vi "Read Power FIFO Direct Dispatch.vi"(7 "Release Lock":bool=TRUE, 8 "error in (no error)":errorcluster, 9 "Timeout (ms)":i32=100, 10 "Power Waveform In":T1, 11 "CIFTag in":refnum<class "CIFChannels.lvclass">) -> (0 "error out":errorcluster, 1 "timed out?":bool, 2 "Power Waveform Out":T1, 3 "CIFTag out":refnum<class "CIF_NIChn_Fifo_Power_DVR.lvclass">, 4 "Header":T2)   [LabVIEW 2021, in "CIF_NIChn_Fifo_Power_DVR.lvclass"]
uses:
  CIF_NIChn_Fifo_Power_DVR.lvclass
  D:/dev/CIF-LVCore/src/Channels/CIFChannels/CIFChannels.lvclass
  D:/dev/CIF-LVCore/src/Channels/CIF_NIChn/NIChn/CIF_NIChn.lvclass
  ChannelCommon/typedef/FIFO Header.ctl
  CIFChannels/CIFChannels.lvclass
  ChannelCommon/typedef/Datatype Power Waveform.ctl
  CIFChannels/CIFChannels.lvclass/CIFChannels.ctl
  NIChn/CIF_NIChn.lvclass/CIF_NIChn.ctl
  CIF_NIChn_Fifo_Power_DVR.lvclass/CIF_NIChn_Fifo_Power_DVR.ctl
  ChannelCommon/CIFFIFO/CIFfifo.lvclass/CIFfifo.ctl
  NIChn/Accessors/Read CIF Channel.vi
  NIChn/SubVIs/Check Disconnect.vi
  <vilib>/CIFChannels/Top Level/Read Variable Length U8 Array.vi
  NIChn/Accessors/Write CIF Channel.vi
  SubVIs/Unflatten.vi
  CIFChannels/Accessors/Read Channel State.vi
  CIFChannels/Accessors/Read Direction.vi
  CIFChannels/Accessors/Write Channel State.vi
  CIFChannels/Accessors/Read Disconnect Behavior.vi
  <vilib>/CIFChannels/Top Level/Read Variable Length U8 Array.vi/81056090-23cf-424a-a716-29db01c8ef1b.vi
  <vilib>/CIFChannels/Top Level/Read Variable Length U8 Array.vi/6610cd62-0a6d-4591-8fd4-6453482a4bc1.vi
  <vilib>/CIFChannels/Top Level/Read Variable Length U8 Array.vi/93d598b0-524b-4f76-9570-a74a86ef2c6f.vi
  ChannelCommon/CIFFIFO/Accessors/Write Timeout.vi
  ChannelCommon/CIFFIFO/Flatten/DVR Unflatten.vi
  ChannelCommon/CIFFIFO/Accessors/Read Header.vi
  ChannelCommon/CIFFIFO/Accessors/Write Header.vi
  <vilib>/CIFChannels/Top Level/Read Variable Length U8 Array.vi/81056090-23cf-424a-a716-29db01c8ef1b.vi/4bc1c15b-36ab-481f-b8dd-c64075ce723a.vi
  <vilib>/CIFChannels/Top Level/Read Variable Length U8 Array.vi/81056090-23cf-424a-a716-29db01c8ef1b.vi/d83cb72b-7713-41fc-a3d1-682de79cf574.vi
  <vilib>/CIFChannels/SubVIs/Get dll Path.vi
  <vilib>/CIFChannels/Top Level/Read Variable Length U8 Array.vi/6610cd62-0a6d-4591-8fd4-6453482a4bc1.vi/c28b0ead-42ad-4072-80a2-aca7f2bd7ce3.vi
  <vilib>/CIFChannels/Top Level/Read Variable Length U8 Array.vi/93d598b0-524b-4f76-9570-a74a86ef2c6f.vi/4bc1c15b-36ab-481f-b8dd-c64075ce723a.vi
  <vilib>/CIFChannels/Top Level/Read Variable Length U8 Array.vi/93d598b0-524b-4f76-9570-a74a86ef2c6f.vi/d83cb72b-7713-41fc-a3d1-682de79cf574.vi
  ChannelCommon/Utilities/Unflatten Header.vi
  CIFCore/Common/Utilities/Add Error.vi
  CIFCore/Common/Utilities/Append Error Location.vi
  NIChn/CIF_NIChn.lvclass
  ChannelCommon/ChannelCommon.lvlib
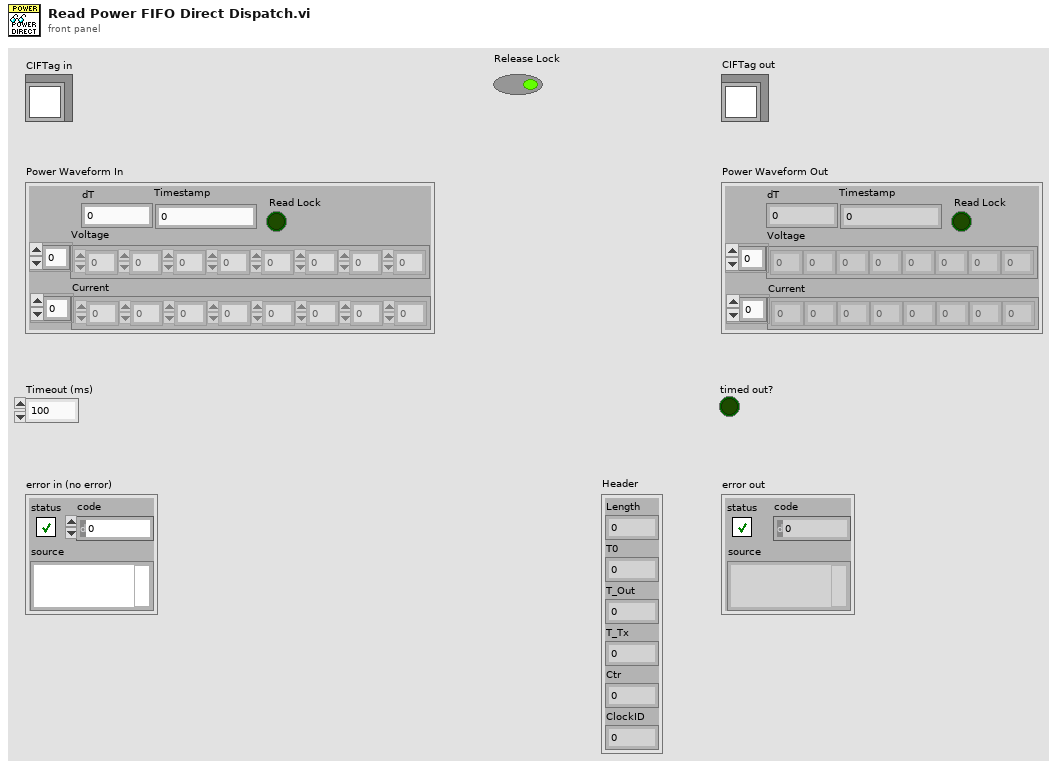
[diagram p1: front panel]
types:
  T1 = typedef "ChannelCommon.lvlib/Datatype Power Waveform.ctl" = cluster{"Voltage":dbl[], "Current":dbl[], "dT":dbl, "Timestamp":u64, "Read Lock":bool}
  T2 = typedef "ChannelCommon.lvlib/FIFO Header.ctl" = cluster{"Length":u64, "T0":u64, "T_Out":u64, "T_Tx":u64, "Ctr":u64, "ClockID":u8}
  T3 = typedef "ChannelCommon.lvlib/Datatype Waveform.ctl" = cluster{"measurement":dbl[], "dT":dbl, "Timestamp":u64, "Read Lock":bool}
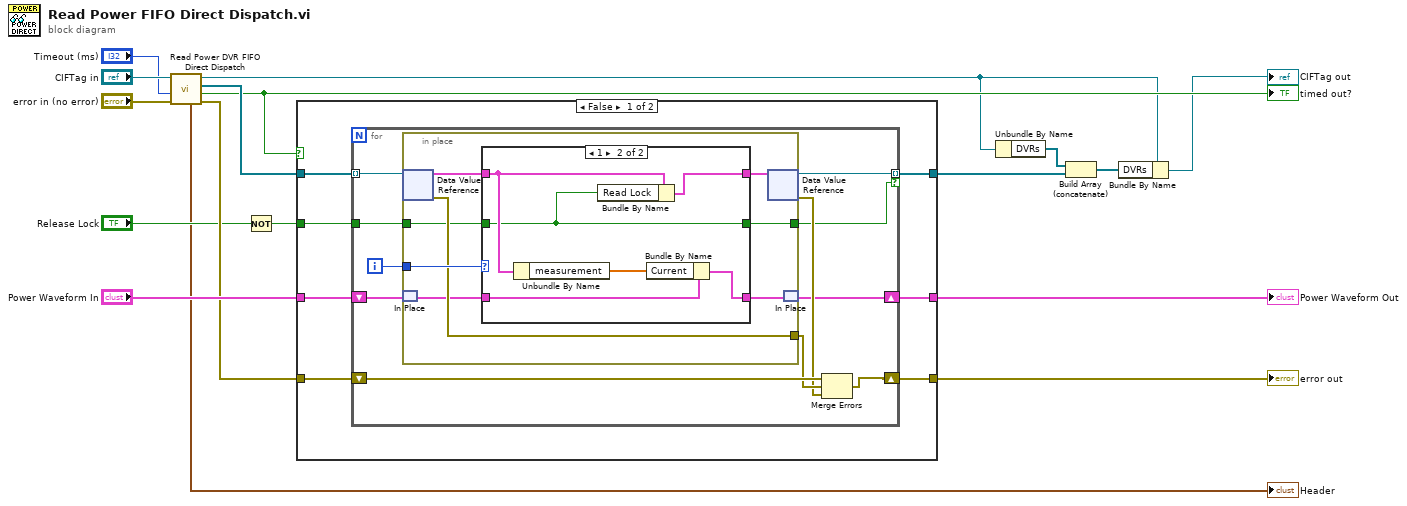
[diagram p0: block diagram]
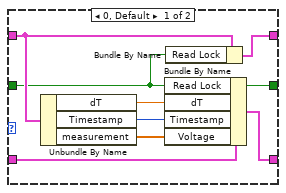
[diagram p2: hidden frame]
diagram:
  n1 = call "Read Power DVR FIFO Direct Dispatch.vi"("error in (no error)"="error in (no error)", "Timeout (ms)"="Timeout (ms)", "CIFTag in"="CIFTag in") -> ("error out"=w14:errorcluster, "timed out?"=w8:bool, "Data Out"=w13:refnum<data-value>[], "CIFTag out"=w4:refnum<class "CIF_NIChn_Fifo_Power_DVR.lvclass">, "Header"=→"Header":T2)  [unwired: 4 in]
  "timed out?" <- w8
  n2 = Not(x="Release Lock") -> (.not. x?=w11:bool)
  n3 = case shown="False" w8 {
    tunnel: w14 -> [w22 w60]
    tunnel: w13 -> [w24 w58]
    tunnel: [w19 w60] -> w9
    tunnel: "Power Waveform In" -> [w23 w59]
    tunnel: w11 -> [w21 _]
    tunnel: [w20 w59] -> w10
    tunnel: [w18 w58] -> w2
    frame False {
      n4 = for {
        tunnel: w24 -> [w35] mode=indexing
        shift-right: [w30] -> w19
        shift-left: w22 -> [w33]
        shift-right: [w25] -> w20
        shift-left: w23 -> [w26]
        tunnel: w21 -> [w29]
        tunnel: [w28] -> w18 mode=indexing if=w27
        i -> [w34]
        n5 = in-place {
          in-place-border: w34 -> [w43]
          in-place-border: [w42] -> w32
          in-place-border: w29 -> [w40]
          in-place-border: [w38] -> w27
          n6 = in-place-dvr #1(w35) -> (w41:T3, w42:errorcluster)
          n7 = in-place-match #2(w26) -> (w37:T1)
          n8 = case shown="1" w43 {
            tunnel: w41 -> [w46 w54]
            tunnel: w37 -> [w51 w57]
            tunnel: [w50 w56] -> w36
            tunnel: w40 -> [w44 w52]
            tunnel: [w45 w53] -> w39
            tunnel: [w44 w52] -> w38
            frame 0, Default {
              n9 = Unbundle By Name(w46) -> ("dT"=w47:dbl, "Timestamp"=w48:u64, "measurement"=w49:dbl[])
              n10 = Bundle By Name(cluster=w51, "Read Lock"=w44, "dT"=w47, "Timestamp"=w48, "Voltage"=w49) -> (w50:T1)
              n11 = Bundle By Name(cluster=w46, "Read Lock"=w44) -> (w45:T3)
            }
            frame 1 {
              n12 = Unbundle By Name(w54) -> ("measurement"=w55:dbl[])
              n13 = Bundle By Name(cluster=w54, "Read Lock"=w52) -> (w53:T3)
              n14 = Bundle By Name(cluster=w57, "Current"=w55) -> (w56:T1)
            }
          }
          n15 = in-place-dvr #1(w39) -> (w28:refnum<data-value>, w31:errorcluster)
          n16 = in-place-match #2(w36) -> (w25:T1)
        }
        n17 = Merge Errors(w33, w32, w31) -> (w30:errorcluster)
      }
    }
    frame True {
    }
  }
  "error out" <- w9
  "Power Waveform Out" <- w10
  n18 = Unbundle By Name(w4) -> ("DVRs"=w3:refnum<data-value>[])
  n19 = Build Array (concatenate)(w3, w2) -> (w1:refnum<data-value>[])
  n20 = Bundle By Name(cluster=w4, "DVRs"=w1) -> (→"CIFTag out":refnum<class "CIF_NIChn_Fifo_Power_DVR.lvclass">)
